vi "compute_init_param.vi"(8 "Current Position (decimicrons)":dbl, 10 "Target Pulse Duration (ms)":dbl, 11 "Target Position (decimicrons)":dbl) -> (1 "Acceleration (decimicrons/s2)":dbl, 2 "Velocity (decimicrons/s)":dbl, 3 "Distance (decimicrons)":dbl)   [LabVIEW 2014]
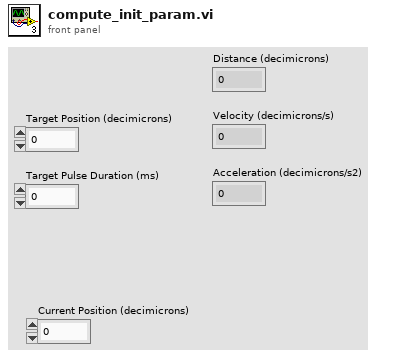
[diagram p1: front panel]
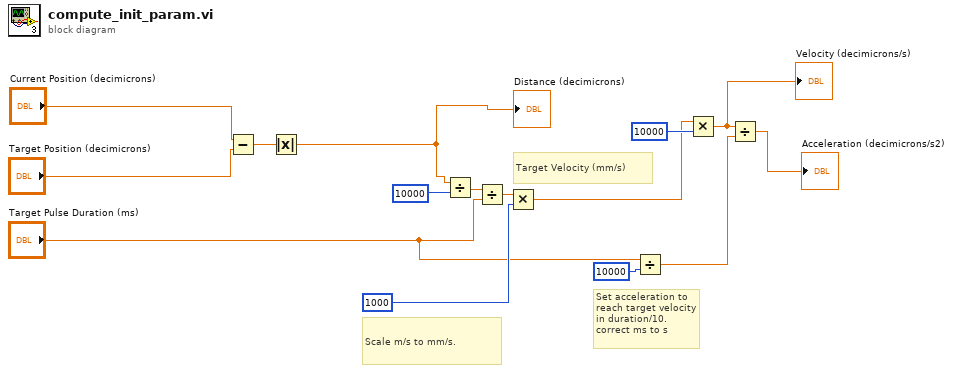
[diagram p0: block diagram]
diagram:
  # "Scale m/s to mm/s."
  # "Target Velocity (mm/s)"
  # "Set acceleration to reach target velocity in duration/10.  correct ms to s"
  n1 = Subtract(x="Current Position (decimicrons)", y="Target Position (decimicrons)") -> (x-y=w4:dbl)
  n2 = Absolute Value(x=w4) -> (abs(x)=w3:dbl)
  "Distance (decimicrons)" <- w3
  n3 = Divide(x=w3, y=10000) -> (x/y=w6:dbl)
  n4 = Divide(x=w6, y="Target Pulse Duration (ms)") -> (x/y=w9:dbl)
  n5 = Multiply(x=w9, y=1000) -> (x*y=w10:dbl)
  n6 = Divide(x="Target Pulse Duration (ms)", y=10000) -> (x/y=w13:dbl)
  n7 = Multiply(x=w10, y=10000) -> (x*y=w14:dbl)
  "Velocity (decimicrons/s)" <- w14
  n8 = Divide(x=w14, y=w13) -> (x/y=→"Acceleration (decimicrons/s2)":dbl)
